vi "NF WF1973_74 BURS Ncyc.vi"(5 "Set(Auto)":bool, 6 "Read(F)":bool, 7 "Mark(1)":dbl=1.0 min=0.5 max=999999.5 step=0.5 format="%.1f", 8 "error in (no error)":errorcluster caption="Error IN", 9 "Set Mark(Input)":u16(ring) items=["Input", "Minimum", "Maximum"], 10 "Ch(Ch1)":bool, 11 "VISAsession":refnum<visa-resource-name>) -> (0 "error out":errorcluster caption="Error OUT", 2 "Query Mark":dbl min=0.0 max=100.0 format="%.1f", 3 "CopyVISAsession":refnum<visa-resource-name>)   [LabVIEW 2010]
panel:
  # "Choose\nInput"
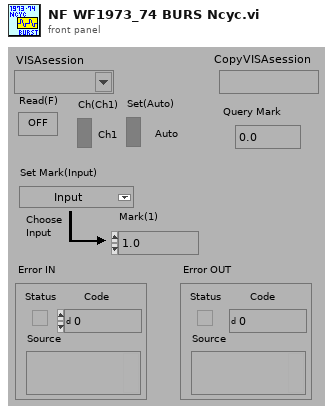
[diagram p1: front panel]
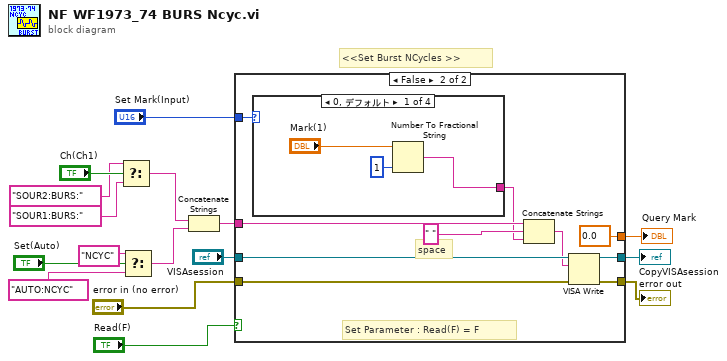
[diagram p0: block diagram]
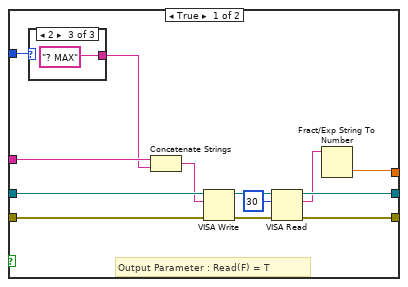
[diagram p2: hidden frame]
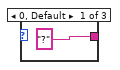
[diagram p3: hidden frame]
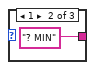
[diagram p4: hidden frame]
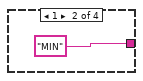
[diagram p5: hidden frame]
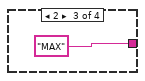
[diagram p6: hidden frame]
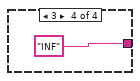
[diagram p7: hidden frame]
diagram:
  # "<<Set Burst NCycles >>"
  n1 = Select(t="SOUR2:BURS:" ("文字列"), s="Ch(Ch1)", f="SOUR1:BURS:" ("文字列")) -> (s? t:f=w3:string)
  n2 = Select(t="NCYC", s="Set(Auto)", f="AUTO:NCYC") -> (s? t:f=w1:string)
  n3 = Concatenate Strings(w3, w1) -> (w4:string)
  n4 = case shown="FALSE" "Read(F)" {
    tunnel: "VISAsession" -> [w29 w42]
    tunnel: [w26 w40] -> w15
    tunnel: [w25 w41] -> w14
    tunnel: "error in (no error)" -> [w24 w36]
    tunnel: w4 -> [w22 w37]
    tunnel: [w19 0.0] -> w11
    tunnel: "Set Mark(Input)" -> [w18 w35]
    frame True {
      # "Output Parameter : Read(F) = T"
      n5 = case shown="2" w18 {
        tunnel: ["?" ("形式文字列") "? MIN" ("形式文字列") "? MAX" ("形式文字列")] -> w17
        frame 0, Default {
        }
        frame 1 {
        }
        frame 2 {
        }
      }
      n6 = Concatenate Strings(w22, w17) -> (w21:string)
      n7 = VISA Write(VISA resource name=w29, write buffer=w21, error in (no error)=w24) -> (VISA resource name out=w27:refnum<visa-resource-name>, error out=w28:errorcluster)  [unwired: 1 out]
      n8 = VISA Read(VISA resource name=w27, byte count=u32 30 ("バイトカウント（0）"), error in (no error)=w28) -> (VISA resource name out=w26:refnum<visa-resource-name>, read buffer=w20:string, error out=w25:errorcluster)  [unwired: 1 out]
      n9 = Fract/Exp String To Number(string=w20) -> (number=w19:dbl)  [unwired: 3 in, 1 out]
    }
    frame False {
      # "space"
      # "Set Parameter : Read(F) = F"
      n10 = case shown="0, デフォルト" w35 {
        tunnel: [w43 "MIN" ("文字列") "MAX" ("文字列") "INF" ("文字列")] -> w34
        frame 0, Default {
          n11 = Number To Fractional String(number="Mark(1)", precision (6)=i16 1 ("精度 (6)")) -> (F-format string=w43:string)  [unwired: 2 in]
        }
        frame 1 {
        }
        frame 2 {
        }
        frame 3 {
        }
      }
      n12 = Concatenate Strings(w37, " ", w34) -> (w39:string)
      n13 = VISA Write(VISA resource name=w42, write buffer=w39, error in (no error)=w36) -> (VISA resource name out=w40:refnum<visa-resource-name>, error out=w41:errorcluster)  [unwired: 1 out]
    }
  }
  "error out" <- w14
  "CopyVISAsession" <- w15
  "Query Mark" <- w11
